vi "readTree.vi"(8 "Fehler (Eingang, kein Fehler)":errorcluster, 10 "Tree ref":refnum<vi>, 11 "Data out (Eingang)":T1={"Report.lvclass"=refnum, "Norm"="", "last State"=enum."Initialize", "Norm ID"=0, "parameter"=[], "EMTestCWS500N.lvclass"=refnum, "CEG4500.lvclass"=refnum, "Tektronix RSA5106A.lvclass"=refnum, "erfolgreich"=FALSE, "log"="", "Kommentar"="", "Device Enum"=enum."emTestCWS500N", "Test Enum"=enum."HF-Felder", "debug"=FALSE, "tab"=enum."Hauptmenü", "ESD Pistol.lvclass"=refnum, "SubPnl Refnum"=refnum, "TabCtl Refnum"=refnum, "ButtonsEinblenden?"=FALSE, "VKey"=enum."ASCII"}) -> (0 "error out":errorcluster, 3 "Data out (Ausgang)":T1={"Report.lvclass"=refnum, "Norm"="", "last State"=enum."Initialize", "Norm ID"=0, "parameter"=[], "EMTestCWS500N.lvclass"=refnum, "CEG4500.lvclass"=refnum, "Tektronix RSA5106A.lvclass"=refnum, "erfolgreich"=FALSE, "log"="", "Kommentar"="", "Device Enum"=enum."emTestCWS500N", "Test Enum"=enum."HF-Felder", "debug"=FALSE, "tab"=enum."Hauptmenü", "ESD Pistol.lvclass"=refnum, "SubPnl Refnum"=refnum, "TabCtl Refnum"=refnum, "ButtonsEinblenden?"=FALSE, "VKey"=enum."ASCII"})   [LabVIEW 2013, in "TreeRepresentation.lvlib"]
doc: "Baumstruktur mit den Prüfdaten aus dem Reiter \"Prüfdaten\" zurücklesen"
uses:
  lib/TreeRepresentation.lvlib
  Main/controls/Data.ctl
  classes/Datastructure/Report/Report.lvclass
  classes/Devices/emTestCWS500N/EMTestCWS500N.lvclass
  classes/Devices/CEG4500/CEG4500.lvclass
  classes/Devices/Tektronix RSA5106A/Tektronix RSA5106A.lvclass
  ESD Pistol.lvclass
  Main/controls/State.ctl
  classes/Devices/DeviceInterface/Devices.ctl
  classes/Tests/TestInterface/Tests.ctl
  Tabs.ctl
  <vilib>/event_ctls.llb/eventvkey.ctl
  classes/Datastructure/Norm/Norm.lvclass
  classes/Datastructure/Test/Test.lvclass
  classes/Datastructure/Image/img.lvclass
  classes/Datastructure/Setup/Setup.lvclass
  classes/Datastructure/Device/Device.lvclass
panel:
  in  "columns":u32
  out "Report.lvclass":refnum<class "Report.lvclass">
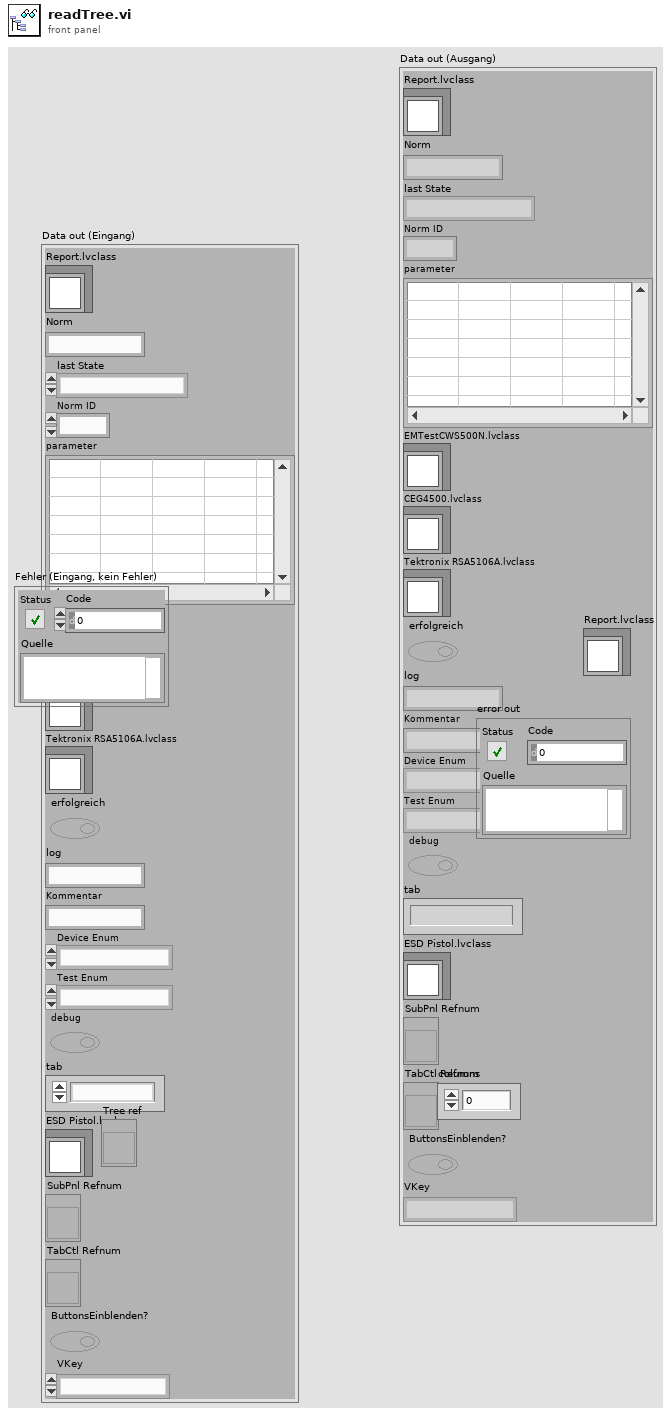
[diagram p1: front panel]
types:
  T1 = typedef "Data.ctl" = cluster{"Report.lvclass":refnum<class "Report.lvclass">, "Norm":string, "last State":T2, "Norm ID":i32, "parameter":string[][], "EMTestCWS500N.lvclass":refnum<class "EMTestCWS500N.lvclass">, "CEG4500.lvclass":refnum<class "CEG4500.lvclass">, "Tektronix RSA5106A.lvclass":refnum<class "Tektronix RSA5106A.lvclass">, "erfolgreich":bool, "log":string, "Kommentar":string, "Device Enum":T3, "Test Enum":T4, "debug":bool, "tab":T5, "ESD Pistol.lvclass":refnum<class "ESD Pistol.lvclass">, "SubPnl Refnum":refnum<vi>, "TabCtl Refnum":refnum<vi>, "ButtonsEinblenden?":bool, "VKey":T6}
  T2 = typedef "State.ctl" = enum16{"create Pdf", "edit Report", "load Report", "save Report", "do Test", "CDN Kalibrierung", "enter Report Parameters", "new Test", "Protokoll", "read Tree", "update Tree", "Fehler", "Initialize", "Wait for Event", "Exit"}
  T3 = typedef "Devices.ctl" = enum16{"unbekannt", "ESD Pistol", "Tektronix RSA5106A", "emTestCWS500N", "CEG-4500"}
  T4 = typedef "Tests.ctl" = enum16{"unbekannt", "Störaussendung", "Burst", "ESD", "Surge", "Spannungseinbruch", "HF-Felder"}
  T5 = typedef "Tabs.ctl" = enum32{"Hauptmenü", "Prüfbericht", "Einstellungen"}
  T6 = typedef "eventvkey.ctl" = enum16{"ASCII", "Enter", "Return", "Shift", "Ctrl", "Alt", "Cmd", "Opt", "Caps", "NumLock", "Clear", "Break", "Up", "Down", "Left", "Right", "Insert", "Delete", "Home", "End", "PageUp", "PageDown", "Escape", "Help", "Pause", "ScrollLock", "F1", "F2", "F3", "F4", "F5", "F6", "F7", "F8", "F9", "F10", "F11", "F12", "F13", "F14", "F15", "F16", "F17", "F18", "F19", "F20", "F21", "F22", "F23", "F24", "Play", "VolumeUp", "VolumeDown", "Mute", "Two Byte Char"}
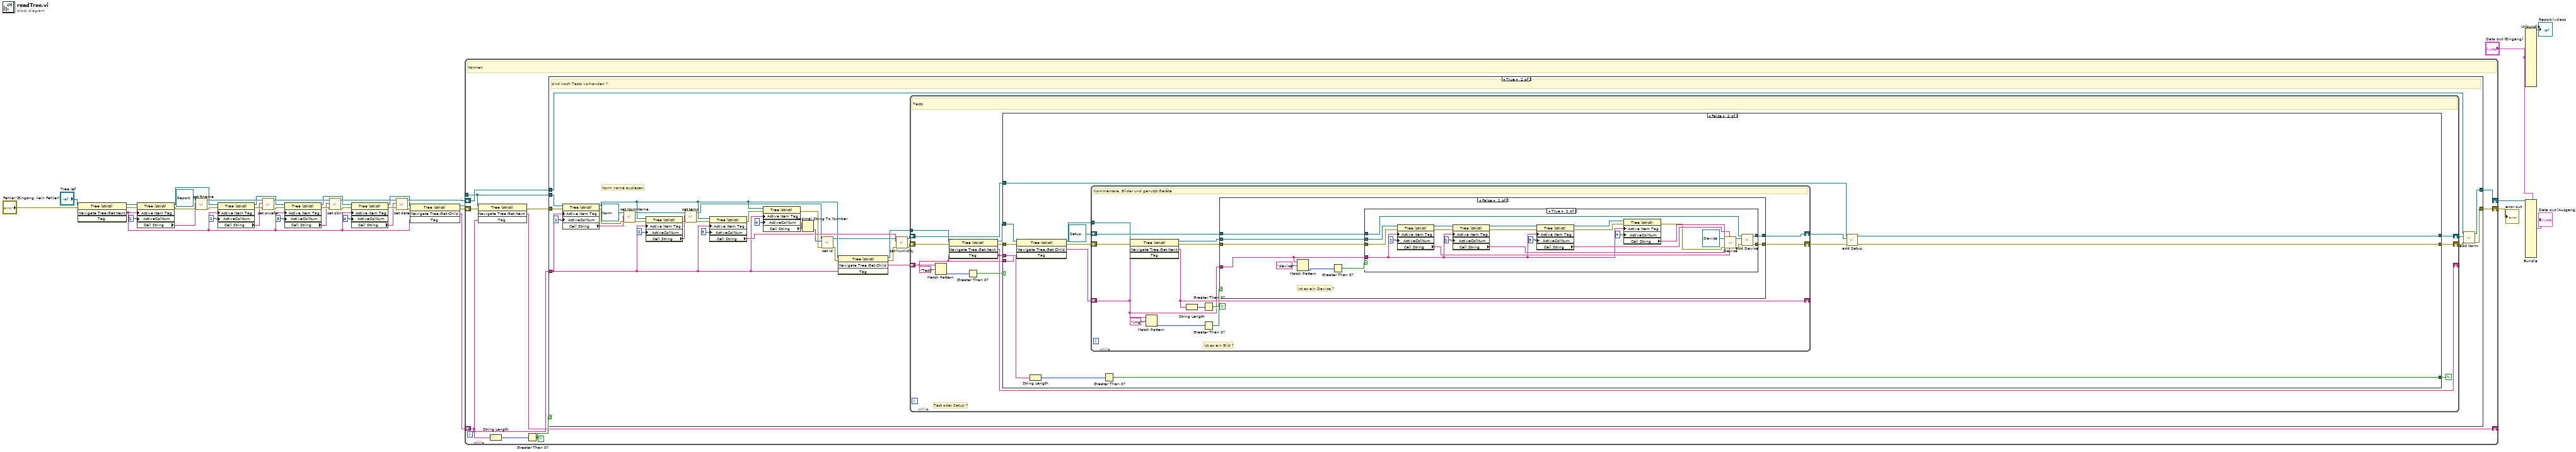
[diagram p0: block diagram]
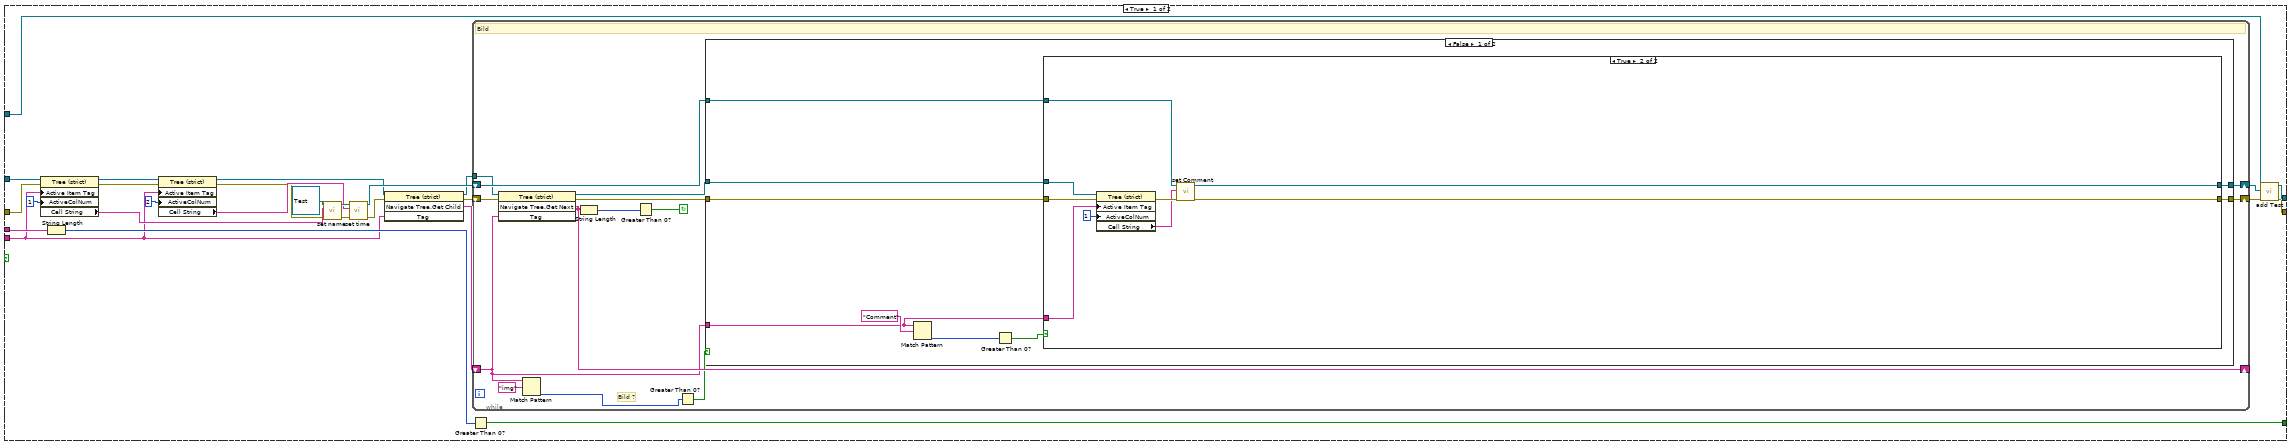
[diagram p3: hidden frame]
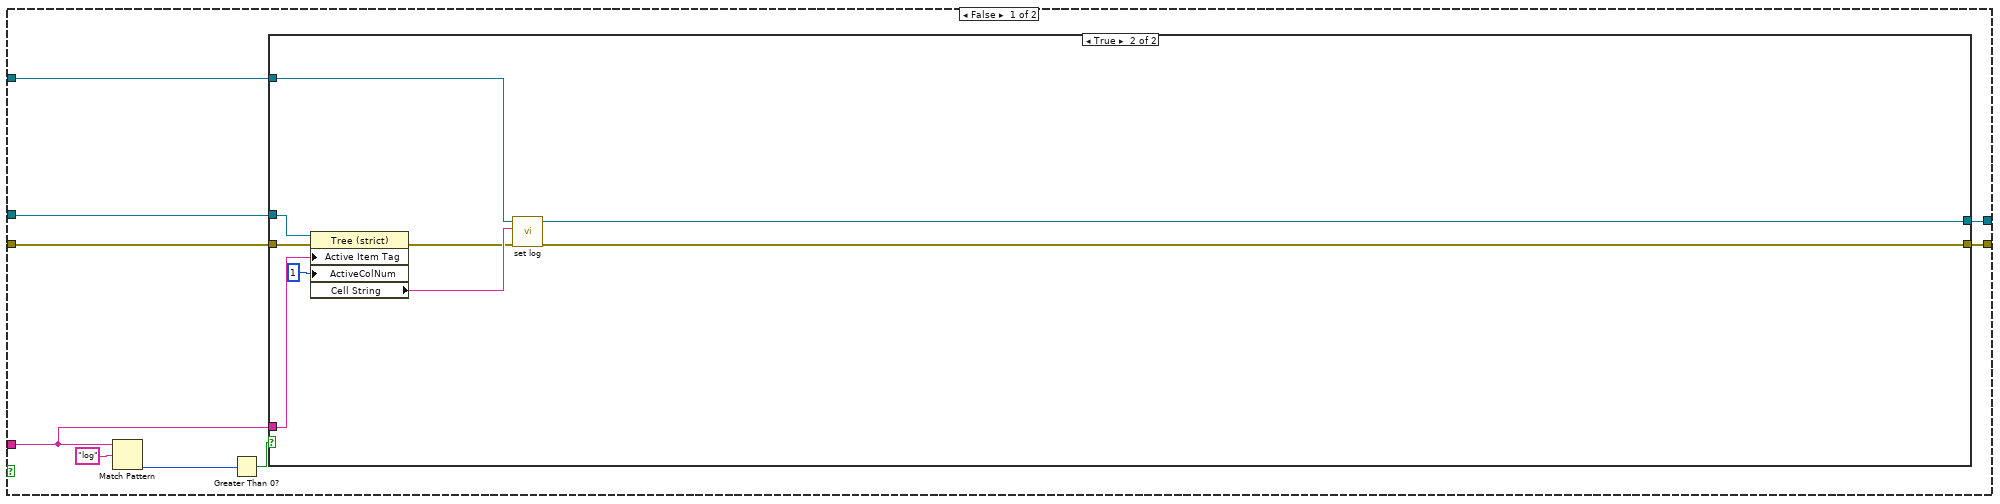
[diagram p4: hidden frame]
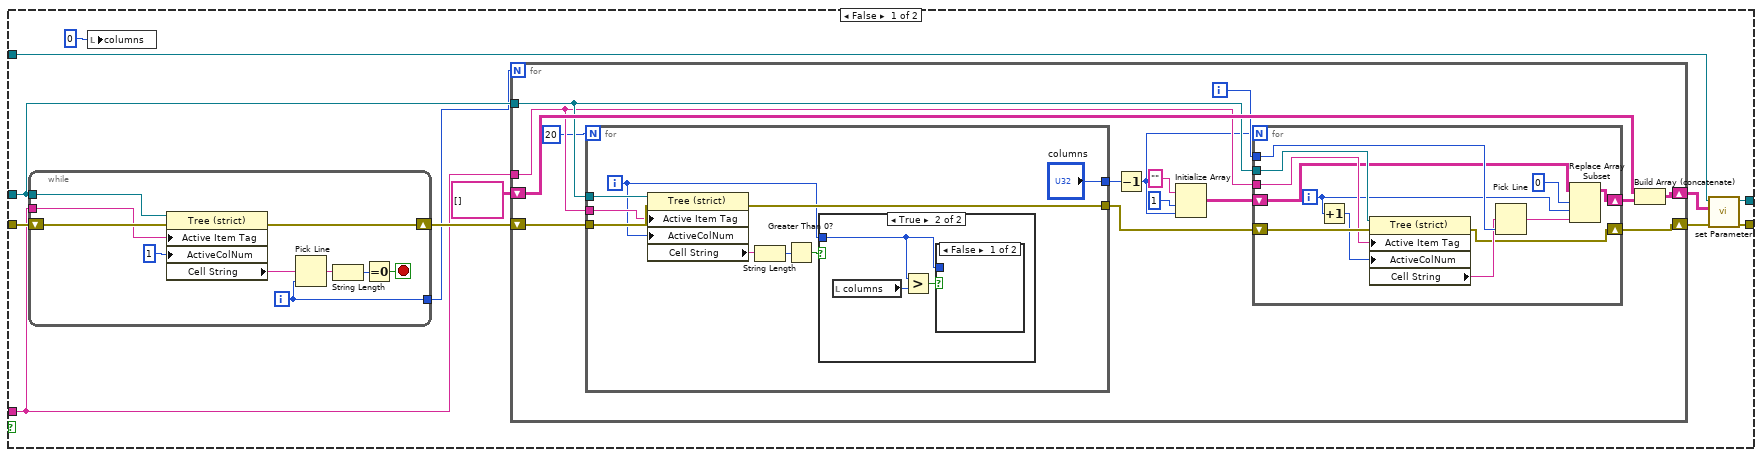
[diagram p5: hidden frame]
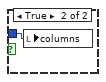
[diagram p7: hidden frame]
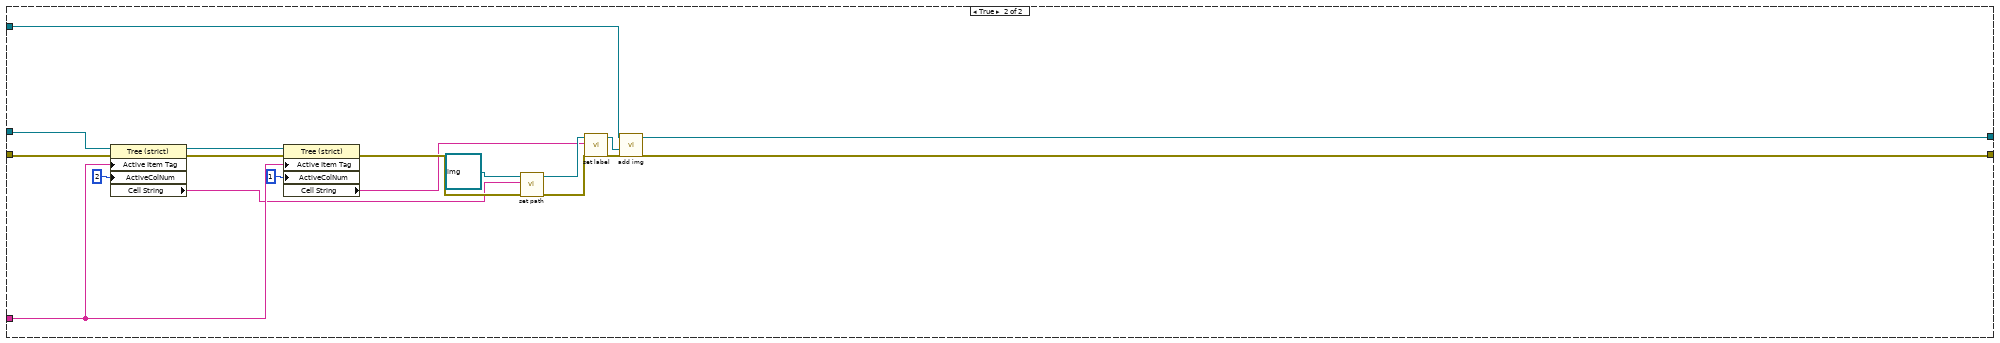
[diagram p8: hidden frame]
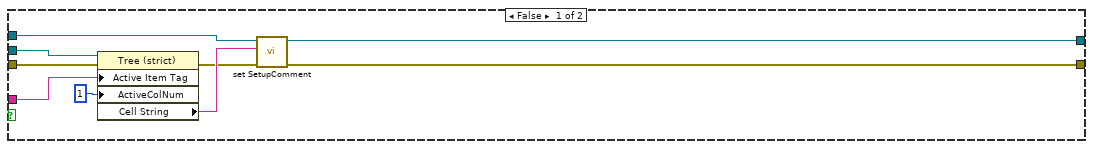
[diagram p9: hidden frame]
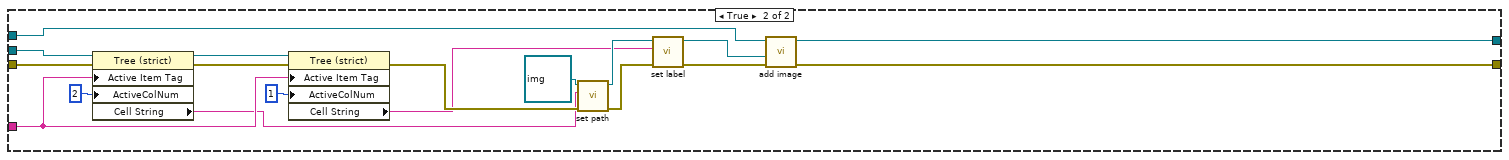
[diagram p10: hidden frame]
diagram:
  n1 = invoke class="Tree (strict)" method="Navigate Tree.Get Next"(reference="Tree ref", error in="Fehler (Eingang, kein Fehler)") -> (reference out=w20:refnum<vi>, error out=w35:errorcluster, "Navigate Tree:Get Next Item"=w5:string)  [unwired: 2 in, 1 out]
  n2 = property class="Tree (strict)"(reference=w20, error in=w35, "Active Item Tag"=w5, "ActiveColNum"=1 ("Aktive Zelle:Nummer der aktiven Spalte")) -> (reference out=w2:refnum<vi>, error out=w31:errorcluster, "Cell String"=w6:string)
  n3 = call-dynamic "set Rname.vi"("error in (no error)"=w31, "Rname"=w6, "Report (Eingang)"=refnum<class "Report.lvclass"> refnum ("Report in")) -> ("error out"=w15:errorcluster, "Report (Ausgang)"=w33:refnum<class "Report.lvclass">)  [unwired: 7 in]
  n4 = property class="Tree (strict)"(reference=w2, error in=w15, "Active Item Tag"=w5, "ActiveColNum"=2 ("Aktive Zelle:Nummer der aktiven Spalte")) -> (reference out=w3:refnum<vi>, error out=w14:errorcluster, "Cell String"=w7:string)
  n5 = call-dynamic "set pruefer.vi"("error in (no error)"=w14, "pruefer"=w7, "Report in"=w33) -> ("error out"=w13:errorcluster, "Report out"=w32:refnum<class "Report.lvclass">)  [unwired: 7 in]
  n6 = property class="Tree (strict)"(reference=w3, error in=w13, "Active Item Tag"=w5, "ActiveColNum"=3 ("Aktive Zelle:Nummer der aktiven Spalte")) -> (reference out=w4:refnum<vi>, error out=w12:errorcluster, "Cell String"=w8:string)
  n7 = call-dynamic "set obnr.vi"("error in (no error)"=w12, "obnr"=w8, "Report in"=w32) -> ("error out"=w11:errorcluster, "Report out"=w23:refnum<class "Report.lvclass">)  [unwired: 7 in]
  n8 = property class="Tree (strict)"(reference=w4, error in=w11, "Active Item Tag"=w5, "ActiveColNum"=4 ("Aktive Zelle:Nummer der aktiven Spalte")) -> (reference out=w1:refnum<vi>, error out=w10:errorcluster, "Cell String"=w9:string)
  n9 = call-dynamic "set date.vi"("error in (no error)"=w10, "date"=w9, "Report (Eingang)"=w23) -> ("error out"=w21:errorcluster, "Report (Ausgang)"=w22:refnum<class "Report.lvclass">)  [unwired: 7 in]
  n10 = invoke class="Tree (strict)" method="Navigate Tree.Get Child"(reference=w1, error in=w21, "Tag"=w5) -> (reference out=w37:refnum<vi>, error out=w34:errorcluster, "Navigate Tree:Get Child"=w36:string)  [unwired: 1 in, 1 out]
  n11 = while {
    tunnel: w37 -> [w43]
    shift-right: [w46] -> w30
    shift-left: w22 -> [w47]
    shift-right: [w44] -> w28
    shift-left: w34 -> [w42]
    shift-right: [w40] -> _
    shift-left: w36 -> [w41]
    stop <- w45 continue-if-true
    # "Normen"
    n12 = invoke class="Tree (strict)" method="Navigate Tree.Get Next"(reference=w43, error in=w42, "Tag"=w41) -> (error out=w39:errorcluster, "Navigate Tree:Get Next Item"=w40:string)  [unwired: 1 in, 2 out]
    n13 = String Length(string=w41) -> (length=w48:i32)
    n14 = Greater Than 0?(x=w48) -> (x > 0?=w45:bool)
    n15 = case shown="True" w45 {
      tunnel: w43 -> [_ w84]
      tunnel: w47 -> [w50 w51]
      tunnel: [w50 w53] -> w46
      tunnel: w41 -> [_ w62]
      tunnel: [w49 w54] -> w44
      tunnel: w39 -> [w49 w80]
      frame False {
      }
      frame True {
        # "Norm name auslesen"
        # "sind noch Tests vorhanden ?"
        n16 = property class="Tree (strict)"(reference=w84, error in=w80, "Active Item Tag"=w62, "ActiveColNum"=1) -> (reference out=w64:refnum<vi>, error out=w81:errorcluster, "Cell String"=w77:string)
        n17 = call-dynamic "set NormName.vi"("error in (no error)"=w81, "name"=w77, "Norm (Eingang)"=refnum<class "Norm.lvclass"> refnum ("Test (Eingang)")) -> ("error out"=w72:errorcluster, "Norm (Ausgang)"=w75:refnum<class "Norm.lvclass">)  [unwired: 7 in]
        n18 = property class="Tree (strict)"(reference=w64, error in=w72, "Active Item Tag"=w62, "ActiveColNum"=2 ("Aktive Zelle:Nummer der aktiven Spalte")) -> (error out=w71:errorcluster, "Cell String"=w67:string)  [unwired: 1 out]
        n19 = call-dynamic "set temp.vi"("error in (no error)"=w71, "temp"=w67, "Norm (Eingang)"=w75) -> ("error out"=w70:errorcluster, "Norm (Ausgang)"=w57:refnum<class "Norm.lvclass">)  [unwired: 7 in]
        n20 = property class="Tree (strict)"(reference=w64, error in=w70, "Active Item Tag"=w62, "ActiveColNum"=3 ("Aktive Zelle:Nummer der aktiven Spalte")) -> (error out=w65:errorcluster, "Cell String"=w66:string)  [unwired: 1 out]
        n21 = property class="Tree (strict)"(reference=w64, error in=w65, "Active Item Tag"=w62, "ActiveColNum"=4 ("Aktive Zelle:Nummer der aktiven Spalte")) -> (error out=w59:errorcluster, "Cell String"=w61:string)  [unwired: 1 out]
        n22 = Decimal String To Number(string=w61) -> (number=w60:i32)  [unwired: 2 in, 1 out]
        n23 = call-dynamic "set id.vi"("error in (no error)"=w59, "id"=w60, "Test (Eingang)"=w57) -> ("error out"=w58:errorcluster, "Test (Ausgang)"=w56:refnum<class "Norm.lvclass">)  [unwired: 7 in]
        n24 = invoke class="Tree (strict)" method="Navigate Tree.Get Child"(reference=w64, error in=w58, "Tag"=w62) -> (reference out=w79:refnum<vi>, error out=w63:errorcluster, "Navigate Tree:Get Child"=w78:string)  [unwired: 1 in, 1 out]
        n25 = call-dynamic "set humidity.vi"("error in (no error)"=w63, "humidity"=w66, "Test (Eingang)"=w56) -> ("error out"=w74:errorcluster, "Test (Ausgang)"=w73:refnum<class "Norm.lvclass">)  [unwired: 7 in]
        n26 = while "While-Schleife" {
          tunnel: w79 -> [w97]
          shift-right: [w94] -> w82
          shift-left: w73 -> [w95]
          shift-right: [w92] -> w52
          shift-left: w74 -> [w93]
          shift-right: [w91] -> _
          shift-left: w78 -> [w87]
          stop <- w96 continue-if-true
          # "Test oder Setup ?"
          # "Tests"
          n27 = Match Pattern(string=w87, regular expression="Test" ("Regulärer Ausdruck")) -> (offset past match=w86:i32)  [unwired: 1 in, 3 out]
          n28 = invoke class="Tree (strict)" method="Navigate Tree.Get Next"(reference=w97, error in=w93, "Tag"=w87) -> (reference out=w90:refnum<vi>, error out=w89:errorcluster, "Navigate Tree:Get Next Item"=w91:string)  [unwired: 1 in, 1 out]
          n29 = Greater Than 0?(x=w86) -> (x > 0?=w85:bool)
          n30 = case shown="False" w85 {
            tunnel: [w123 w268] -> w96
            tunnel: w95 -> [w122 w259]
            tunnel: [w121 w258] -> w94
            tunnel: [w120 w257] -> w92
            tunnel: w91 -> [w110 w264]
            tunnel: w90 -> [w109 w261]
            tunnel: w89 -> [w108 w260]
            tunnel: w87 -> [w102 w263]
            frame True {
              n31 = property class="Tree (strict)"(reference=w109, error in=w108, "Active Item Tag"=w102, "ActiveColNum"=1 ("Aktive Zelle:Nummer der aktiven Spalte")) -> (reference out=w104:refnum<vi>, error out=w103:errorcluster, "Cell String"=w106:string)
              n32 = String Length(string=w110) -> (length=w124:i32)
              n33 = property class="Tree (strict)"(reference=w104, error in=w103, "Active Item Tag"=w102, "ActiveColNum"=2 ("Aktive Zelle:Nummer der aktiven Spalte")) -> (reference out=w100:refnum<vi>, error out=w99:errorcluster, "Cell String"=w101:string)
              n34 = call-dynamic "set name.vi"("error in (no error)"=w99, "name"=w106, "Test (Eingang)"=refnum<class "Test.lvclass"> refnum ("Segment (Eingang)")) -> ("error out"=w116:errorcluster, "Test (Ausgang)"=w119:refnum<class "Test.lvclass">)  [unwired: 7 in]
              n35 = call-dynamic "set time.vi"("error in (no error)"=w116, "time"=w101, "Test (Eingang)"=w119) -> ("error out"=w114:errorcluster, "Test (Ausgang)"=w117:refnum<class "Test.lvclass">)  [unwired: 7 in]
              n36 = invoke class="Tree (strict)" method="Navigate Tree.Get Child"(reference=w100, error in=w114, "Tag"=w102) -> (reference out=w112:refnum<vi>, error out=w113:errorcluster, "Navigate Tree:Get Child"=w111:string)  [unwired: 1 in, 1 out]
              n37 = Greater Than 0?(x=w124) -> (x > 0?=w123:bool)
              n38 = while {
                shift-right: [w137] -> w98
                shift-left: w117 -> [w138]
                shift-right: [w134] -> w115
                shift-left: w113 -> [w133]
                tunnel: w112 -> [w132]
                shift-right: [w131] -> _
                shift-left: w111 -> [w125]
                stop <- w135 continue-if-true
                # "Bild ?"
                # "Bild"
                n39 = invoke class="Tree (strict)" method="Navigate Tree.Get Next"(reference=w132, error in=w133, "Tag"=w125) -> (reference out=w129:refnum<vi>, error out=w130:errorcluster, "Navigate Tree:Get Next Item"=w131:string)  [unwired: 1 in, 1 out]
                n40 = Match Pattern(string=w125, regular expression="img" ("Regulärer Ausdruck")) -> (offset past match=w127:i32)  [unwired: 1 in, 3 out]
                n41 = String Length(string=w131) -> (length=w136:i32)
                n42 = Greater Than 0?(x=w136) -> (x > 0?=w135:bool)
                n43 = Greater Than 0?(x=w127) -> (x > 0?=w126:bool)
                n44 = case shown="False" w126 {
                  tunnel: w138 -> [w147 w251]
                  tunnel: [w146 w250] -> w137
                  tunnel: [w145 w244] -> w134
                  tunnel: w130 -> [w144 w243]
                  tunnel: w129 -> [w143 w242]
                  tunnel: w125 -> [w141 w241]
                  frame False {
                    n45 = Match Pattern(string=w141, regular expression="Comment" ("Regulärer Ausdruck")) -> (offset past match=w140:i32)  [unwired: 1 in, 3 out]
                    n46 = Greater Than 0?(x=w140) -> (x > 0?=w139:bool)
                    n47 = case shown="True" w139 {
                      tunnel: w147 -> [w153 w236]
                      tunnel: [w148 w235] -> w146
                      tunnel: [w149 w233] -> w145
                      tunnel: w144 -> [w151 w232]
                      tunnel: w143 -> [w152 w231]
                      tunnel: w141 -> [w150 w228]
                      frame False {
                        n48 = Match Pattern(string=w150, regular expression="log" ("Regulärer Ausdruck")) -> (offset past match=w155:i32)  [unwired: 1 in, 3 out]
                        n49 = Greater Than 0?(x=w155) -> (x > 0?=w154:bool)
                        n50 = case shown="True" w154 {
                          tunnel: w153 -> [w164 w227]
                          tunnel: w152 -> [w162 w226]
                          tunnel: w151 -> [w161 w225]
                          tunnel: w150 -> [w159 w224]
                          tunnel: [w167 w220] -> w149
                          tunnel: [w168 w219] -> w148
                          frame False {
                            n51 = while {
                              tunnel: w162 -> [w218]
                              shift-right: [w216] -> w160
                              shift-left: w161 -> [w217]
                              tunnel: w159 -> [w214]
                              tunnel: [w209] -> w158
                              i -> [w209]
                              stop <- w210 stop-if-true
                              n52 = property class="Tree (strict)"(reference=w218, error in=w217, "Active Item Tag"=w214, "ActiveColNum"=1 ("Aktive Zelle:Nummer der aktiven Spalte")) -> (error out=w216:errorcluster, "Cell String"=w211:string)  [unwired: 1 out]
                              n53 = Pick Line(multi-line string=w211, line index=w209) -> (output string=w213:string)  [unwired: 1 in]
                              n54 = String Length(string=w213) -> (length=w212:i32)
                              n55 = Equal To 0?(x=w212) -> (x = 0?=w210:bool)
                            }
                            n56 = local write "columns"(u32 0 ("columns")) -> ()
                            n57 = for {
                              N: w158 -> [_]
                              tunnel: w162 -> [w173]
                              tunnel: w159 -> [w172]
                              shift-right: [w183] -> w166
                              shift-left: string[][] [] -> [w181]
                              shift-right: [w182] -> w165
                              shift-left: w160 -> [w175]
                              i -> [w176]
                              n58 = for {
                                N: 20 -> [_]
                                tunnel: w175 -> [w192]
                                tunnel: [w191] -> w174
                                tunnel: w173 -> [w190]
                                tunnel: w172 -> [w189]
                                tunnel: ["columns"] -> w170
                                i -> [w184]
                                n59 = property class="Tree (strict)"(reference=w190, error in=w192, "Active Item Tag"=w189, "ActiveColNum"=w184) -> (error out=w191:errorcluster, "Cell String"=w188:string)  [unwired: 1 out]
                                n60 = String Length(string=w188) -> (length=w186:i32)
                                n61 = Greater Than 0?(x=w186) -> (x > 0?=w187:bool)
                                n62 = case shown="True" w187 {
                                tunnel: w184 -> [_ w194]
                                frame False {
                                }
                                frame True {
                                n63 = local read "columns"() -> (w195:u32)
                                n64 = Greater?(x=w194, y=w195) -> (0:w193:bool)
                                n65 = case shown="False" w193 {
                                tunnel: w194 -> [_ w196]
                                frame False {
                                }
                                frame True {
                                n66 = local write "columns"(w196) -> ()
                                }
                                }
                                }
                                }
                              }
                              n67 = Decrement(x=w170) -> (x-1=w169:u32)
                              n68 = Initialize Array("" ("Element"), 1 ("Dimension"), w169) -> (w177:string[][])
                              n69 = for {
                                N: w169 -> [_]
                                tunnel: w173 -> [w207]
                                tunnel: w172 -> [w206]
                                tunnel: w176 -> [w203]
                                shift-right: [w200] -> w182
                                shift-left: w174 -> [w208]
                                shift-right: [w205] -> w180
                                shift-left: w177 -> [w199]
                                i -> [w197]
                                n70 = Increment(x=w197) -> (x+1=w204:i32)
                                n71 = property class="Tree (strict)"(reference=w207, error in=w208, "Active Item Tag"=w206, "ActiveColNum"=w204) -> (error out=w200:errorcluster, "Cell String"=w202:string)  [unwired: 1 out]
                                n72 = Pick Line(multi-line string=w202, line index=w203) -> (output string=w201:string)  [unwired: 1 in]
                                n73 = Replace Array Subset(array=w199, new element=w201, index (row)=0 ("Deaktivierter Index (Zeile)"), index (col)=w197) -> (w205:string[][])
                              }
                              n74 = Build Array (concatenate)(w181, w180) -> (w183:string[][])
                            }
                            n75 = call-dynamic "set Parameter.vi"("error in (no error)"=w165, "Parameter"=w166, "Test (Eingang)"=w164) -> ("error out"=w167:errorcluster, "Test (Ausgang)"=w168:refnum<class "Test.lvclass">)  [unwired: 7 in]
                          }
                          frame True {
                            n76 = property class="Tree (strict)"(reference=w226, error in=w225, "Active Item Tag"=w224, "ActiveColNum"=1 ("Aktive Zelle:Nummer der aktiven Spalte")) -> (error out=w221:errorcluster, "Cell String"=w222:string)  [unwired: 1 out]
                            n77 = call-dynamic "set log.vi"("error in (no error)"=w221, "log"=w222, "Test (Eingang)"=w227) -> ("error out"=w220:errorcluster, "Test (Ausgang)"=w219:refnum<class "Test.lvclass">)  [unwired: 7 in]
                          }
                        }
                      }
                      frame True {
                        n78 = property class="Tree (strict)"(reference=w231, error in=w232, "Active Item Tag"=w228, "ActiveColNum"=1 ("Aktive Zelle:Nummer der aktiven Spalte")) -> (error out=w234:errorcluster, "Cell String"=w229:string)  [unwired: 1 out]
                        n79 = call-dynamic "set Comment.vi"("error in (no error)"=w234, "Comment"=w229, "Test (Eingang)"=w236) -> ("error out"=w233:errorcluster, "Test (Ausgang)"=w235:refnum<class "Test.lvclass">)  [unwired: 7 in]
                      }
                    }
                  }
                  frame True {
                    n80 = property class="Tree (strict)"(reference=w242, error in=w243, "Active Item Tag"=w241, "ActiveColNum"=2 ("Aktive Zelle:Nummer der aktiven Spalte")) -> (reference out=w249:refnum<vi>, error out=w248:errorcluster, "Cell String"=w239:string)
                    n81 = property class="Tree (strict)"(reference=w249, error in=w248, "Active Item Tag"=w241, "ActiveColNum"=1 ("Aktive Zelle:Nummer der aktiven Spalte")) -> (error out=w247:errorcluster, "Cell String"=w238:string)  [unwired: 1 out]
                    n82 = call-dynamic "set path.vi"("error in (no error)"=w247, "path"=w239, "img (Eingang)"=refnum<class "img.lvclass"> refnum ("img.lvclass")) -> ("error out"=w246:errorcluster, "img (Ausgang)"=w253:refnum<class "img.lvclass">)  [unwired: 7 in]
                    n83 = call-dynamic "set label.vi"("error in (no error)"=w246, "label"=w238, "img (Eingang)"=w253) -> ("error out"=w245:errorcluster, "img (Ausgang)"=w252:refnum<class "img.lvclass">)  [unwired: 7 in]
                    n84 = call-dynamic "add img.vi"("error in (no error)"=w245, "img.lvclass"=w252, "Test (Eingang)"=w251) -> ("error out"=w244:errorcluster, "Test (Ausgang)"=w250:refnum<class "Test.lvclass">)  [unwired: 6 in]
                  }
                }
              }
              n85 = call-dynamic "add Test.vi"("error in (no error)"=w115, "Test.lvclass"=w98, "Test Eingang"=w122) -> ("error out"=w120:errorcluster, "Test Ausgang"=w121:refnum<class "Norm.lvclass">)  [unwired: 7 in]
            }
            frame False {
              n86 = invoke class="Tree (strict)" method="Navigate Tree.Get Child"(reference=w261, error in=w260, "Tag"=w263) -> (reference out=w266:refnum<vi>, error out=w267:errorcluster, "Navigate Tree:Get Child"=w265:string)  [unwired: 1 in, 1 out]
              n87 = String Length(string=w264) -> (length=w269:i32)
              n88 = while {
                shift-right: [w282] -> w255
                shift-left: refnum<class "Setup.lvclass"> refnum ("Setup.lvclass") -> [w283]
                shift-right: [w279] -> w256
                shift-left: w267 -> [w278]
                tunnel: w266 -> [w277]
                shift-right: [w276] -> _
                shift-left: w265 -> [w270]
                stop <- w280 continue-if-true
                # "ist es ein Bild ?"
                # "Kommentare, Bilder und genutzt Geräte"
                n89 = invoke class="Tree (strict)" method="Navigate Tree.Get Next"(reference=w277, error in=w278, "Tag"=w270) -> (reference out=w274:refnum<vi>, error out=w275:errorcluster, "Navigate Tree:Get Next Item"=w276:string)  [unwired: 1 in, 1 out]
                n90 = Match Pattern(string=w270, regular expression="img" ("Regulärer Ausdruck")) -> (offset past match=w272:i32)  [unwired: 1 in, 3 out]
                n91 = String Length(string=w276) -> (length=w281:i32)
                n92 = Greater Than 0?(x=w281) -> (x > 0?=w280:bool)
                n93 = Greater Than 0?(x=w272) -> (x > 0?=w271:bool)
                n94 = case shown="False" w271 {
                  tunnel: w283 -> [w289 w330]
                  tunnel: [w290 w329] -> w282
                  tunnel: [w288 w328] -> w279
                  tunnel: w275 -> [w292 w337]
                  tunnel: w274 -> [w291 w336]
                  tunnel: w270 -> [w285 w335]
                  frame False {
                    # "ist es ein Device ?"
                    n95 = Match Pattern(string=w285, regular expression="device" ("Regulärer Ausdruck")) -> (offset past match=w287:i32)  [unwired: 1 in, 3 out]
                    n96 = Greater Than 0?(x=w287) -> (x > 0?=w284:bool)
                    n97 = case shown="True" w284 {
                      tunnel: w292 -> [w300 w325]
                      tunnel: w291 -> [w301 w324]
                      tunnel: [w293 w316] -> w290
                      tunnel: w289 -> [w296 w315]
                      tunnel: [w294 w313] -> w288
                      tunnel: w285 -> [w297 w308]
                      frame False {
                        n98 = property class="Tree (strict)"(reference=w301, error in=w300, "Active Item Tag"=w297, "ActiveColNum"=1 ("Aktive Zelle:Nummer der aktiven Spalte")) -> (error out=w295:errorcluster, "Cell String"=w298:string)  [unwired: 1 out]
                        n99 = call-dynamic "set SetupComment.vi"("error in (no error)"=w295, "Comment"=w298, "Setup (Eingang)"=w296) -> ("error out"=w294:errorcluster, "Setup (Ausgang)"=w293:refnum<class "Setup.lvclass">)  [unwired: 7 in]
                      }
                      frame True {
                        n100 = property class="Tree (strict)"(reference=w324, error in=w325, "Active Item Tag"=w308, "ActiveColNum"=2 ("Aktive Zelle:Nummer der aktiven Spalte")) -> (reference out=w322:refnum<vi>, error out=w321:errorcluster, "Cell String"=w303:string)
                        n101 = property class="Tree (strict)"(reference=w322, error in=w321, "Active Item Tag"=w308, "ActiveColNum"=1 ("Aktive Zelle:Nummer der aktiven Spalte")) -> (reference out=w320:refnum<vi>, error out=w319:errorcluster, "Cell String"=w302:string)
                        n102 = property class="Tree (strict)"(reference=w320, error in=w319, "Active Item Tag"=w308, "ActiveColNum"=3 ("Aktive Zelle:Nummer der aktiven Spalte")) -> (reference out=w309:refnum<vi>, error out=w310:errorcluster, "Cell String"=w305:string)
                        n103 = property class="Tree (strict)"(reference=w309, error in=w310, "Active Item Tag"=w308, "ActiveColNum"=4 ("Active Cell:Active Column Number")) -> (error out=w304:errorcluster, "Cell String"=w306:string)  [unwired: 1 out]
                        n104 = call-dynamic "Device.vi"("Model"=w303, "last calibration"=w305, "error in (no error)"=w304, "Hersteller"=w302, "serial"=w306, "Device Eingang"=refnum<class "Device.lvclass"> refnum) -> ("error out"=w314:errorcluster, "Device Ausgang"=w312:refnum<class "Device.lvclass">)  [unwired: 4 in]
                        n105 = call-dynamic "add Device.vi"("error in (no error)"=w314, "Device.lvclass"=w312, "Setup Eingang"=w315) -> ("error out"=w313:errorcluster, "Setup Ausgang"=w316:refnum<class "Setup.lvclass">)  [unwired: 7 in]
                      }
                    }
                  }
                  frame True {
                    n106 = property class="Tree (strict)"(reference=w336, error in=w337, "Active Item Tag"=w335, "ActiveColNum"=2 ("Aktive Zelle:Nummer der aktiven Spalte")) -> (reference out=w341:refnum<vi>, error out=w340:errorcluster, "Cell String"=w333:string)
                    n107 = property class="Tree (strict)"(reference=w341, error in=w340, "Active Item Tag"=w335, "ActiveColNum"=1 ("Aktive Zelle:Nummer der aktiven Spalte")) -> (error out=w339:errorcluster, "Cell String"=w332:string)  [unwired: 1 out]
                    n108 = call-dynamic "set path.vi"("error in (no error)"=w339, "path"=w333, "img (Eingang)"=refnum<class "img.lvclass"> refnum ("img.lvclass")) -> ("error out"=w338:errorcluster, "img (Ausgang)"=w342:refnum<class "img.lvclass">)  [unwired: 7 in]
                    n109 = call-dynamic "set label.vi"("error in (no error)"=w338, "label"=w332, "img (Eingang)"=w342) -> ("error out"=w327:errorcluster, "img (Ausgang)"=w326:refnum<class "img.lvclass">)  [unwired: 7 in]
                    n110 = call-dynamic "add image.vi"("error in (no error)"=w327, "img.lvclass"=w326, "Setup (Eingang)"=w330) -> ("error out"=w328:errorcluster, "Setup (Ausgang)"=w329:refnum<class "Setup.lvclass">)  [unwired: 7 in]
                  }
                }
              }
              n111 = Greater Than 0?(x=w269) -> (x > 0?=w268:bool)
              n112 = call-dynamic "add Setup.vi"("error in (no error)"=w256, "Setup"=w255, "Test Eingang"=w259) -> ("error out"=w257:errorcluster, "Test Ausgang"=w258:refnum<class "Norm.lvclass">)  [unwired: 7 in]
            }
          }
        }
        n113 = call-dynamic "add Norm.vi"("error in (no error)"=w52, "Norm.lvclass"=w82, "Report (Eingang)"=w51) -> ("error out"=w54:errorcluster, "Report (Ausgang)"=w53:refnum<class "Report.lvclass">)  [unwired: 7 in]
      }
    }
  }
  "error out" <- w28
  n114 = Unbundle("Data out (Eingang)") -> ("Report.lvclass"=→"Report.lvclass":refnum<class "Report.lvclass">)  [unwired: 19 out]
  n115 = Bundle(cluster="Data out (Eingang)", "Report.lvclass"=w30) -> (→"Data out (Ausgang)":T1)  [unwired: 19 in]
